vi "circuits-terminal.vi"(4 "Density":dbl=0.01, 5 "GetPOS Y":refnum<vi>, 6 "Diension":dbl=0.1, 7 "GetPOS X":refnum<vi>, 8 "Device in Y":refnum<k24>, 11 "Device in X":refnum<k24>) -> (0 "Device out Y":refnum<k24>, 3 "Device out X":refnum<k24>)   [LabVIEW 2014]
doc: "André Romero - 2019\nandretec@ifsc.usp.br"
uses:
  C:/user-Lab/AndreTec/GITs/andretec/Thorlabs-Vector-Move/kinesisTec/Kinesis/Thorlabs.MotionControl.TCube.DCServoCLI.dll
  kinesisTec/Kinesis/Thorlabs.MotionControl.TCube.DCServoCLI.dll
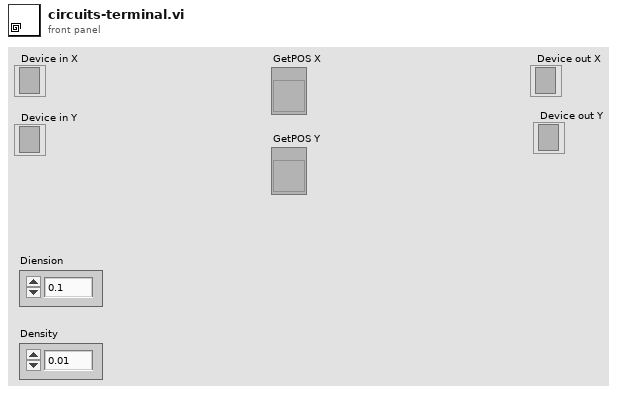
[diagram p1: front panel]
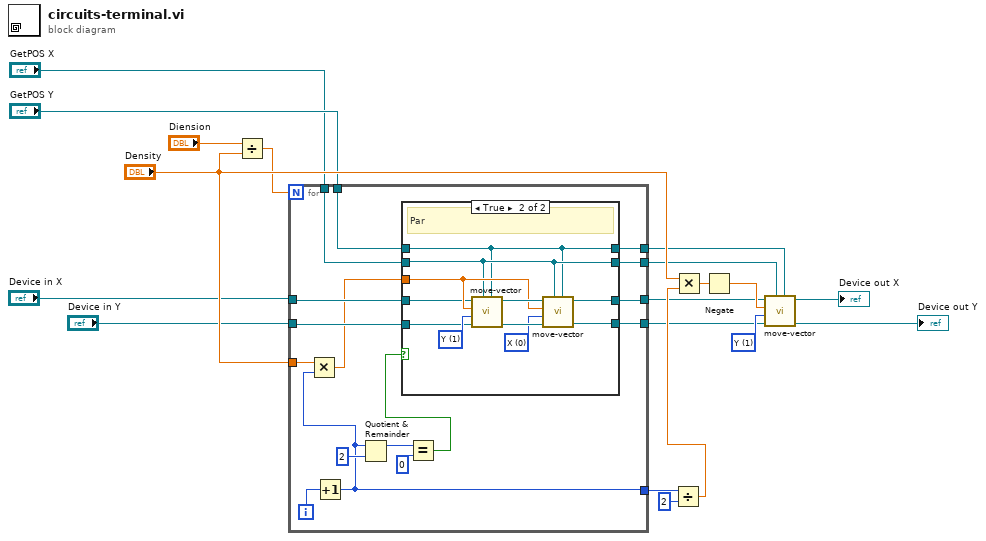
[diagram p0: block diagram]
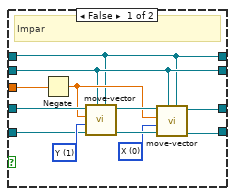
[diagram p2: hidden frame]
diagram:
  w13 = u16 1 items=["X", "Y"] ("X-Y")
  n1 = Divide(x="Diension", y="Density") -> (x/y=w3:dbl)
  n2 = for {
    N: w3 -> [_]
    tunnel: "Device in X" -> [w35]
    tunnel: [w33] -> w9
    tunnel: "Device in Y" -> [w34]
    tunnel: [w32] -> w10
    tunnel: "Density" -> [w24]
    tunnel: "GetPOS X" -> [w26]
    tunnel: "GetPOS Y" -> [w25]
    tunnel: [w22] -> w11
    tunnel: [w21] -> w12
    tunnel: [w20] -> w14
    i -> [w28]
    n3 = Increment(x=w28) -> (x+1=w20:i32)
    n4 = Multiply(x=w24, y=w20) -> (x*y=w23:dbl)
    n5 = Quotient & Remainder(x=w20, y=2) -> (x-y*floor(x/y)=w30:i32)  [unwired: 1 out]
    n6 = Equal?(x=w30, y=0) -> (x = y?=w27:bool)
    n7 = case shown="True" w27 {
      tunnel: w35 -> [w46 w52]
      tunnel: w34 -> [w45 w53]
      tunnel: [w39 w51] -> w33
      tunnel: [w38 w50] -> w32
      tunnel: w23 -> [w44 w54]
      tunnel: w26 -> [w37 w49]
      tunnel: w25 -> [w36 w48]
      tunnel: [w37 w49] -> w22
      tunnel: [w36 w48] -> w21
      frame False {
        w40 = u16 0 items=["X", "Y"] ("X-Y")
        w47 = u16 1 items=["X", "Y"] ("X-Y")
        # "Impar"
        n8 = Negate(x=w44) -> (-x=w41:dbl)
        n9 = call "move-vector.vi"("GetPOS Y"=w36, "GetPOS X"=w37, "Device in Y"=w45, "X-Y"=w47, "Distance"=w41, "Device in X"=w46) -> ("Device out Y"=w42:refnum<k24>, "Device out X"=w43:refnum<k24>)  [unwired: 4 in]
        n10 = call "move-vector.vi"("GetPOS Y"=w36, "GetPOS X"=w37, "Device in Y"=w42, "X-Y"=w40, "Distance"=w41, "Device in X"=w43) -> ("Device out Y"=w38:refnum<k24>, "Device out X"=w39:refnum<k24>)  [unwired: 4 in]
      }
      frame True {
        w55 = u16 0 items=["X", "Y"] ("X-Y")
        w58 = u16 1 items=["X", "Y"] ("X-Y")
        # "Par"
        n11 = call "move-vector.vi"("GetPOS Y"=w48, "GetPOS X"=w49, "Device in Y"=w53, "X-Y"=w58, "Distance"=w54, "Device in X"=w52) -> ("Device out Y"=w56:refnum<k24>, "Device out X"=w57:refnum<k24>)  [unwired: 4 in]
        n12 = call "move-vector.vi"("GetPOS Y"=w48, "GetPOS X"=w49, "Device in Y"=w56, "X-Y"=w55, "Distance"=w54, "Device in X"=w57) -> ("Device out Y"=w50:refnum<k24>, "Device out X"=w51:refnum<k24>)  [unwired: 4 in]
      }
    }
  }
  n13 = Divide(x=w14, y=2) -> (x/y=w16:dbl)
  n14 = Multiply(x="Density", y=w16) -> (x*y=w18:dbl)
  n15 = Negate(x=w18) -> (-x=w19:dbl)
  n16 = call "move-vector.vi"("GetPOS Y"=w12, "GetPOS X"=w11, "Device in Y"=w10, "X-Y"=w13, "Distance"=w19, "Device in X"=w9) -> ("Device out Y"=→"Device out Y":refnum<k24>, "Device out X"=→"Device out X":refnum<k24>)  [unwired: 4 in]
